vi "Set Menu Item Info.vi"(4 "short cut":T1, 5 "Picture":refnum<class "Image.lvclass">, 6 "checked":bool, 7 "item tag":string, 8 "error in (no error)":errorcluster, 9 "enabled":bool, 10 "item name":string, 11 "Menu in":refnum<class "Menu.lvclass">) -> (0 "error out":errorcluster, 3 "Menu out":refnum<class "Menu.lvclass">)   [LabVIEW 2021, in "Menu.lvlib" / "Menu.lvclass"]
uses:
  Menu.lvclass
  Menu.lvclass/Menu.ctl
  <vilib>/Utility/miscctls.llb/LVMapReplaceAction.ctl
  MenuItems.ctl
  <vilib>/Utility/miscctls.llb/LVMenuShortCut.ctl
  Picture2D/src/2DPictureControl/2DPictureControl.lvclass
  Picture2D/src/Picture/Image.lvclass
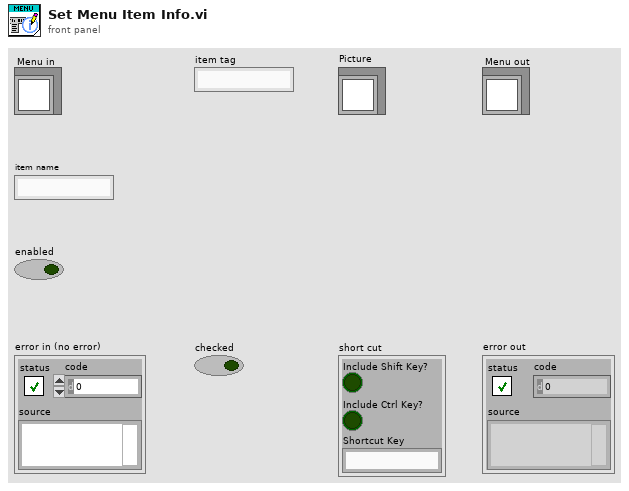
[diagram p1: front panel]
types:
  T1 = typedef "LVMenuShortCut.ctl" = cluster{"Include Shift Key?":bool, "Include Ctrl Key?":bool, "Shortcut Key":string}
  T2 = typedef "Menu.lvlib/Menu.lvclass/MenuItems.ctl" = cluster{"Item Name":string, "Short Cut":T1, "Checked":bool, "Enable":bool, "After item":string, "Item Tags":string[], "Item Names":string[], "Picture":refnum<class "Image.lvclass">, "Hilite Picture":refnum<class "Image.lvclass">, "Displayed":bool}
  T3 = typedef "LVMapReplaceAction.ctl" = enum32{"Modify Entry only if found", "Add or Modify Entry", "Delete Entry"}
  T4 = typedef "Menu.lvlib/Menu.lvclass/Data.ctl" = cluster{"MenuMap":map{string, T2}, "PictRef":refnum<vi>, "MenuSelectionEvent":refnum<user-event>, "TopMenuSpacing":i32, "MenuSpacing":i32, "CloseEvent":refnum<user-event>, "TR_ManageMenuRef":refnum<vi>, "MenuColors":T5, "RTMPath":path, "RTMVIReference":refnum<vi>, "RTMMenuReference":refnum<k9>, "CtlRef":refnum<vi>, "User-Specified Font":refnum<class "Font.lvclass">, "Desired Font":enum16{"User-specified Font", "Application Font", "System Font", "Dialog Font"}, "SubMenuIcon":T6, "SubMenuIconClosed":refnum<class "Picture2D.lvclass">, "SubMenuIconOpened":refnum<class "Picture2D.lvclass">}
  T5 = typedef "Menu.lvlib/Menu.lvclass/MenuColors.ctl" = cluster{"Text":refnum<class "Color.lvclass">, "HiliteText":refnum<class "Color.lvclass">, "Background":refnum<class "Color.lvclass">, "BorderColor":refnum<class "Color.lvclass">, "Hilite":refnum<class "Color.lvclass">}
  T6 = typedef "Menu.lvlib/Menu.lvclass/SubMenuIcon.ctl" = enum16{"LabVIEW", "Windows", "Custom"}
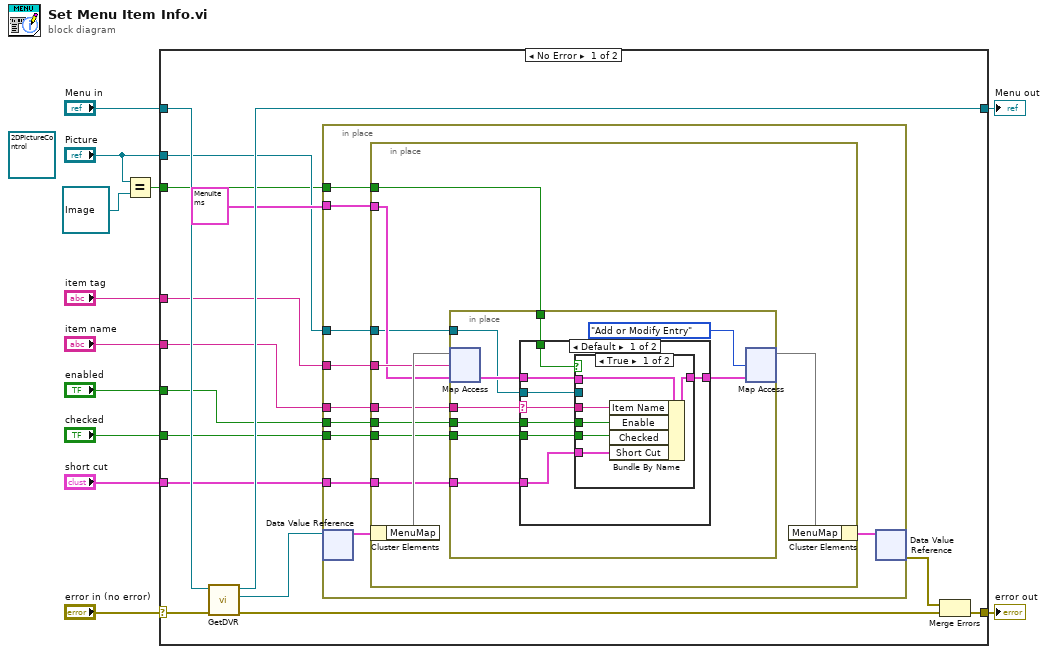
[diagram p0: block diagram]
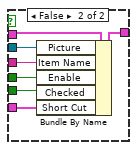
[diagram p2: hidden frame]
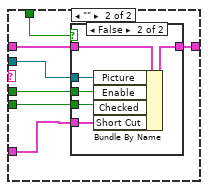
[diagram p3: hidden frame]
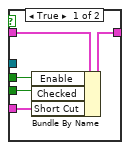
[diagram p4: hidden frame]
diagram:
  (unwired) refnum<class "2DPictureControl.lvclass"> refnum ("Picture")
  (unwired) refnum<class "2DPictureControl.lvclass"> refnum ("Picture")
  n1 = Equal?(x="Picture", y=refnum<class "Image.lvclass"> refnum ("Picture")) -> (x = y?=w1:bool)
  n2 = case shown="No Error" "error in (no error)" {
    selector: "error in (no error)" -> [w27 w97]
    tunnel: [w15 w97] -> w11
    tunnel: [w25 w96] -> w9
    tunnel: "Menu in" -> [w24 w96]
    tunnel: "item name" -> [w21 _]
    tunnel: "enabled" -> [w17 _]
    tunnel: "item tag" -> [w22 _]
    tunnel: "checked" -> [w18 _]
    tunnel: "short cut" -> [w19 _]
    tunnel: "Picture" -> [w16 _]
    tunnel: w1 -> [w13 _]
    frame No Error {
      n3 = call "GetDVR.vi"("error in (no error)"=w27, "Menu in"=w24) -> ("error out"=w26:errorcluster, "DVR"=w23:refnum<data-value>, "Menu out"=w25:refnum<class "Menu.lvclass">)  [unwired: 7 in]
      n4 = in-place {
        in-place-border: w22 -> [w36]
        in-place-border: w21 -> [w34]
        in-place-border: T2 {"Item Name"="", "Short Cut"={"Include Shift Key?"=FALSE, "Include Ctrl Key?"=FALSE, "Shortcut Key"=""}, "Checked"=FALSE, "Enable"=FALSE, "After item"="", "Item Tags"=[], "Item Names"=[], "Picture"=refnum, "Hilite Picture"=refnum, "Displayed"=FALSE} ("Menu") -> [w33]
        in-place-border: w19 -> [w32]
        in-place-border: w18 -> [w31]
        in-place-border: w17 -> [w30]
        in-place-border: w16 -> [w29]
        in-place-border: w13 -> [w28]
        n5 = in-place-dvr #1(w23) -> (w37:T4)  [unwired: 1 out]
        n6 = in-place {
          in-place-border: w36 -> [w46]
          in-place-border: w34 -> [w44]
          in-place-border: w33 -> [w43]
          in-place-border: w32 -> [w42]
          in-place-border: w31 -> [w41]
          in-place-border: w30 -> [w40]
          in-place-border: w29 -> [w39]
          in-place-border: w28 -> [w38]
          n7 = in-place-cluster #2(w37) -> ("MenuMap"=w47:map{string, T2})
          n8 = in-place {
            in-place-border: w44 -> [w55]
            in-place-border: w42 -> [w52]
            in-place-border: w41 -> [w51]
            in-place-border: w40 -> [w50]
            in-place-border: w39 -> [w49]
            in-place-border: w38 -> [w48]
            n9 = in-place-map #3(w47, w46, w43) -> (w54:T2)  [unwired: 1 out]
            n10 = case shown="Default" w55 {
              selector: w55 -> [w62 _]
              tunnel: w54 -> [w64 w84]
              tunnel: [w63 w83] -> w53
              tunnel: w52 -> [w61 w82]
              tunnel: w51 -> [w60 w81]
              tunnel: w50 -> [w59 w80]
              tunnel: w49 -> [w58 w79]
              tunnel: w48 -> [w57 w78]
              frame Default {
                n11 = case shown="True" w57 {
                  tunnel: w64 -> [w70 w77]
                  tunnel: [w69 w76] -> w63
                  tunnel: w62 -> [w68 w75]
                  tunnel: w61 -> [w67 w74]
                  tunnel: w60 -> [w66 w73]
                  tunnel: w59 -> [w65 w72]
                  tunnel: w58 -> [_ w71]
                  frame True {
                    n12 = Bundle By Name(cluster=w70, "Item Name"=w68, "Enable"=w65, "Checked"=w66, "Short Cut"=w67) -> (w69:T2)
                  }
                  frame False {
                    n13 = Bundle By Name(cluster=w77, "Picture"=w71, "Item Name"=w75, "Enable"=w72, "Checked"=w73, "Short Cut"=w74) -> (w76:T2)
                  }
                }
              }
              frame "" {
                n14 = case shown="False" w78 {
                  tunnel: w84 -> [w89 w95]
                  tunnel: [w88 w94] -> w83
                  tunnel: w82 -> [w87 w93]
                  tunnel: w81 -> [w86 w92]
                  tunnel: w80 -> [w85 w91]
                  tunnel: w79 -> [_ w90]
                  frame True {
                    n15 = Bundle By Name(cluster=w89, "Enable"=w85, "Checked"=w86, "Short Cut"=w87) -> (w88:T2)
                  }
                  frame False {
                    n16 = Bundle By Name(cluster=w95, "Picture"=w90, "Enable"=w91, "Checked"=w92, "Short Cut"=w93) -> (w94:T2)
                  }
                }
              }
            }
            n17 = in-place-map #3(w53, LVMapReplaceAction."Add or Modify Entry" ("action")) -> (w45:map{string, T2})  [unwired: 2 out]
          }
          n18 = in-place-cluster #2("MenuMap"=w45) -> (w35:T4)
        }
        n19 = in-place-dvr #1(w35) -> (w14:errorcluster)  [unwired: 1 out]
      }
      n20 = Merge Errors(w14, w26) -> (w15:errorcluster)
    }
    frame Error {
    }
  }
  "error out" <- w11
  "Menu out" <- w9
